vi "GetUser.vi"(8 "error in (no error)":errorcluster, 11 "reference in":refnum<class "MES_Base.lvclass">) -> (0 "error out":errorcluster, 1 "LoggedIn":bool, 2 "User":string, 3 "reference in":refnum<class "MES_Base.lvclass">)   [LabVIEW 2022 SP3, in "MES_Base.lvlib" / "MES_Base.lvclass"]
uses:
  MES_Base.lvclass
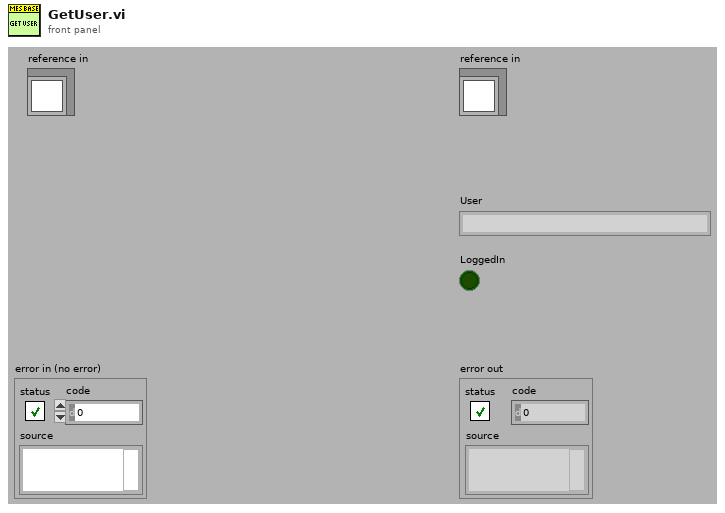
[diagram p1: front panel]
types:
  T1 = typedef "MES_Base.lvlib/MES_Base.lvclass/ObjectAttributes.ctl" = cluster{"Config":T2}
  T2 = typedef "MES_Base.lvlib/MES_Base.lvclass/Config.ctl" = cluster{"WorkflowStep":string}
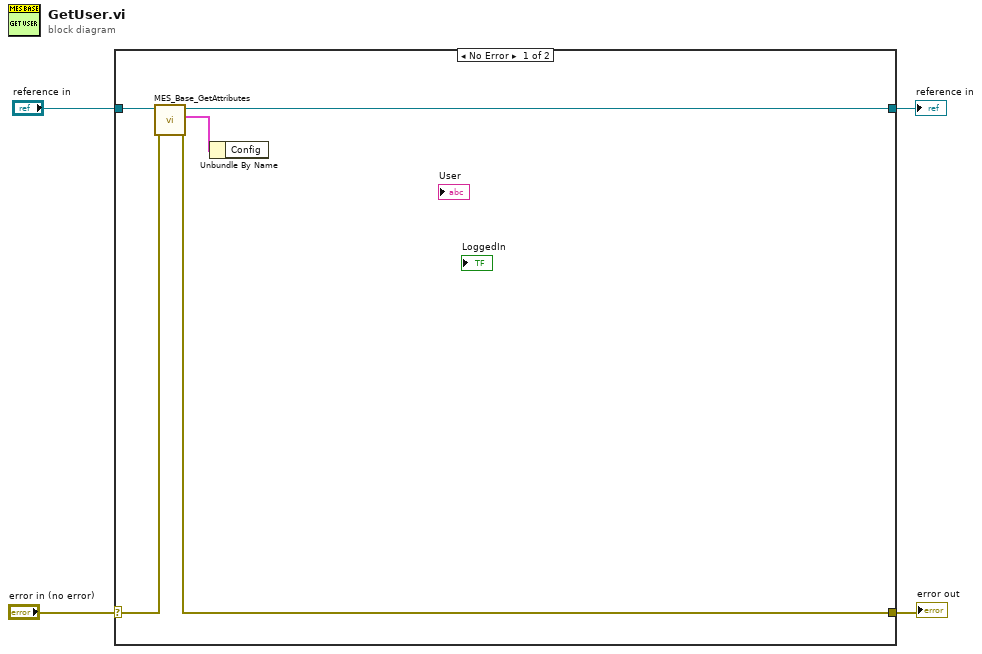
[diagram p0: block diagram]
diagram:
  n1 = case shown="No Error" "error in (no error)" {
    selector: "error in (no error)" -> [w9 w11]
    tunnel: [w7 w11] -> w3
    tunnel: [w5 w10] -> w1
    tunnel: "reference in" -> [w6 w10]
    frame No Error {
      n2 = call "MES_Base_GetAttributes.vi"("error in (no error)"=w9, "reference in"=w6) -> ("error out"=w7:errorcluster, "Data"=w8:T1, "reference out"=w5:refnum<class "MES_Base.lvclass">)  [unwired: 6 in, 1 out]
      n3 = Unbundle By Name(w8) -> ()  [unwired: 1 out]
    }
    frame Error {
    }
  }
  "error out" <- w3
  "reference in" <- w1
